vi "Read Handle.vi"(8 "Error In":errorcluster, 11 "SFTP In":refnum<class "SFTP.lvclass">) -> (0 "Erorr Out":errorcluster, 2 "Handle":u64, 3 "SFTP Out":refnum<class "SFTP.lvclass">)   [LabVIEW 2021, in "Field_RnD_Services_LIBSSH2_Toolkit.lvlib" / "SFTP.lvclass"]
doc: "Gets the memory address for the SFTP struct in the libssh2lv shared library. This value should not be modified and only used with extreme caution."
uses:
  220524-VNA RP FLAT.llb/SFTP.lvclass
  220524-VNA RP FLAT.llb/SFTP.lvclass/SFTP.ctl
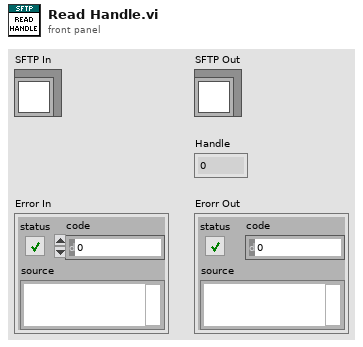
[diagram p1: front panel]
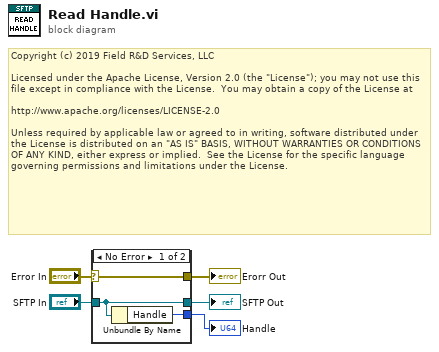
[diagram p0: block diagram]
diagram:
  # "Copyright (c) 2019 Field R&D Services, LLC\n\nLicensed under the Apache License, Version 2.0 (the \"License\"); you may not use this file except in compliance with the License.  You may obtain a copy of the License at\n\nhttp://www.apache.org/licenses/LICENSE-2.0\n\nUnless required by applicable law or agreed to in writing, software distributed under the License is distributed on an \"AS IS\" BASIS, WITHOUT WARRANTIES OR CONDITIONS OF ANY KIND, either express or implied.  See the License for the specific language governing permissions and limitations under the License."
  n1 = case shown="No Error" "Error In" {
    selector: "Error In" -> [w8 w9]
    tunnel: [w8 w9] -> w4
    tunnel: "SFTP In" -> [w7 w10]
    tunnel: [w7 w10] -> w1
    tunnel: [w6 _] -> w3
    frame No Error {
      n2 = Unbundle By Name(w7) -> ("Handle"=w6:u64)
    }
    frame Error {
    }
  }
  "Erorr Out" <- w4
  "Handle" <- w3
  "SFTP Out" <- w1
